vi "GetSetFinalValue.vi"(0 "VISA resource name":refnum<visa-resource-name>, 5 "get/set":T2=enum."set", 7 "Channel Number (1-4)":T1=1 items=["Channel 1"=1, "Channel 2"=2, "Channel 3"=3, "Channel 4"=4], 9 "Set Final Value":dbl min=-200.0 max=300.0 step=1.0 format="%.1f", 11 "error in":errorcluster) -> (4 "VISA resource name out":refnum<visa-resource-name>, 6 "Get Final value":dbl, 8 "8800 response":string, 15 "error out":errorcluster)   [LabVIEW 2023, in "Thermotron 8800.lvlib"]
doc: "FVAL\nCommand name: Send or load final value\nCommand type: Program status; edit from hold\nDescription: The query command asks the 8800 for the current interval’s final value for channel n (1 through 4). The 8800 sends a decimal value for the selected channel. The edit from\nhold operation command temporarily changes the current interval’s final value. NOTE:\nWhen not running a program, the command returns the manual mode new setpoint.\nSyntax: FVALn?\nWhere n is any control channel (1 through 4).\nData type: Decimal\nQuery example 1: FVAL2?\n8800 response: 25.0 (The control channel 2 final value for the current interval is 25.0.)\nQuery example 2: FVAL1?\n8800 response: 50.0 (In manual mode, the channel 1 new setpoint is 50.0.)\nOperation example: FVAL1,-33\n8800 response: 0 (The 8800 loads -33 as the final value for control channel 1.)"
uses:
  Thermotron 8800.lvlib
  Private/get set.ctl
  Private/AnalogInputChannelNumber 1-4.ctl
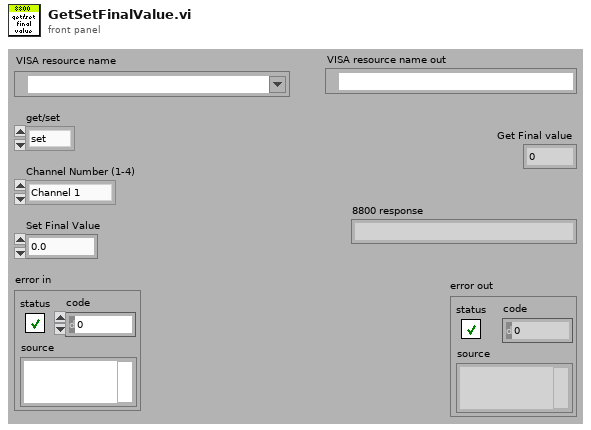
[diagram p1: front panel]
types:
  T1 = typedef "Thermotron 8800.lvlib/AnalogInputChannelNumber 1-4.ctl" = u16
  T2 = typedef "Thermotron 8800.lvlib/get set.ctl" = enum16{"get", "set"}
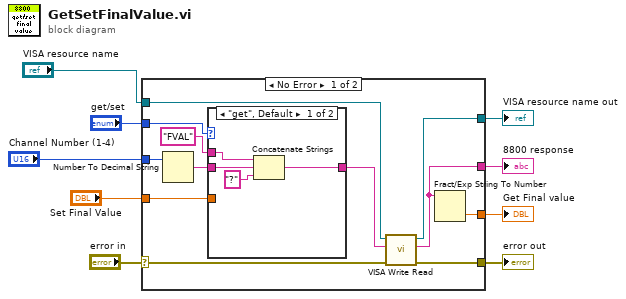
[diagram p0: block diagram]
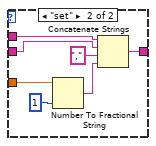
[diagram p2: hidden frame]
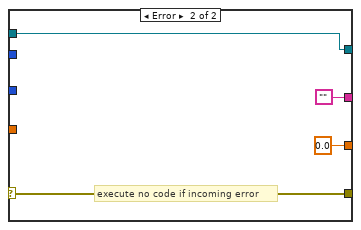
[diagram p3: hidden frame]
diagram:
  n1 = case shown="No Error" "error in" {
    selector: "error in" -> [w19 w36]
    tunnel: [w17 w36] -> w8
    tunnel: [w18 w35] -> w7
    tunnel: "VISA resource name" -> [w20 w35]
    tunnel: "get/set" -> [w16 _]
    tunnel: [w11 ""] -> w4
    tunnel: "Set Final Value" -> [w14 _]
    tunnel: "Channel Number (1-4)" -> [w13 _]
    tunnel: [w10 0.0] -> w1
    frame No Error {
      n2 = Number To Decimal String(number=w13) -> (decimal integer string=w12:string)  [unwired: 1 in]
      n3 = case shown="\"get\", Default" w16 {
        tunnel: "FVAL" ("8800 Command") -> [w24 w32]
        tunnel: [w25 w31] -> w21
        tunnel: w14 -> [_ w29]
        tunnel: w12 -> [w22 w28]
        frame "get", Default {
          n4 = Concatenate Strings(w24, w22, "?" ("8800 Command")) -> (w25:string)
        }
        frame "set" {
          n5 = Number To Fractional String(number=w29, precision (6)=i16 1) -> (F-format string=w26:string)  [unwired: 2 in]
          n6 = Concatenate Strings(w32, w28, "," ("string"), w26) -> (w31:string)
        }
      }
      n7 = call "VISA Write Read.vi"("error in (no error)"=w19, "8800 Command"=w21, "VISA Refnum in"=w20) -> ("error out"=w17:errorcluster, "read buffer"=w11:string, "VISA Refnum out"=w18:refnum<visa-resource-name>)  [unwired: 6 in]
      n8 = Fract/Exp String To Number(string=w11) -> (number=w10:dbl)  [unwired: 3 in, 1 out]
    }
    frame Error {
      # "execute no code if incoming error"
    }
  }
  "VISA resource name out" <- w7
  "error out" <- w8
  "8800 response" <- w4
  "Get Final value" <- w1
